vi "change_image_type.vi"(8 "error in (no error)":errorcluster, 10 "target image type":T1 items=["Grayscale (U8)", "Grayscale (I16)", "Grayscale (SGL)", "Complex (CSG)", "RGB (U32)", "HSL (U32)", "RGB (U64)", "Grayscale (U16)"], 11 "Image in":refnum<class "Image.lvclass">) -> (0 "error out":errorcluster, 3 "Image out":refnum<class "Image.lvclass">)   [LabVIEW 2010, in "Image.lvclass"]
uses:
  Image.lvclass
  storage_mode.ctl
  ErrorController/ErrorController/class_data.vi
  <vilib>/vision/NI_Vision_Development_Module.lvlib
  ErrorController/ErrorController/ErrorController.lvclass
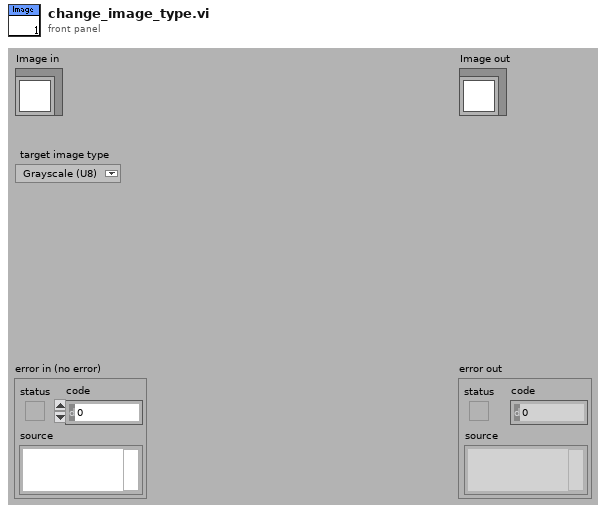
[diagram p1: front panel]
types:
  T1 = typedef "Image Type" = u32
  T2 = typedef "Image.lvclass/storage_mode.ctl" = enum16{"RAM", "disk"}
  T3 = typedef "IMAQ Image.ctl" = refnum<image>
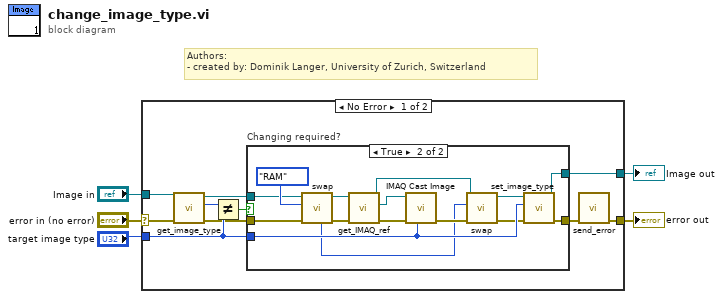
[diagram p0: block diagram]
diagram:
  # "Authors: \n- created by: Dominik Langer, University of Zurich, Switzerland"
  n1 = case shown="No Error" "error in (no error)" {
    selector: "error in (no error)" -> [w15 w34]
    tunnel: [w7 w34] -> w4
    tunnel: [w12 w33] -> w2
    tunnel: "Image in" -> [w13 w33]
    tunnel: "target image type" -> [w11 _]
    frame No Error {
      n2 = call-dynamic "get_image_type.vi"("error in (no error)"=w15, "Image.lvclass in"=w13) -> ("error out"=w10:errorcluster, "Image Type"=w14:T1, "Image.lvclass out"=w9:refnum<class "Image.lvclass">)  [unwired: 6 in, 1 out]
      n3 = Not Equal?(x=w14, y=w11) -> (x != y?=w8:bool)
      n4 = case "Changing required?" shown="True" w8 {
        tunnel: [w16 w32] -> w6
        tunnel: [w17 w29] -> w12
        tunnel: w11 -> [_ w28]
        tunnel: w10 -> [w16 w27]
        tunnel: w9 -> [w17 w24]
        frame False {
        }
        frame True {
          n5 = call-dynamic "swap.vi"("error in (no error)"=w27, "storage type target"=storage_mode."RAM", "Image in"=w24) -> ("error out"=w26:errorcluster, "Image out"=w23:refnum<class "Image.lvclass">, "previous storage mode"=w20:T2)  [unwired: 6 in]
          n6 = call-dynamic "get_IMAQ_ref.vi"("error in (no error)"=w26, "Image.lvclass in"=w23) -> ("error out"=w31:errorcluster, "Image"=w30:T3, "Image.lvclass out"=w19:refnum<class "Image.lvclass">)  [unwired: 5 in, 2 out]
          n7 = call "IMAQ Cast Image"("Image Type"=w28, "error in (no error)"=w31, "Image Src"=w30) -> ("error out"=w22:errorcluster)  [unwired: 7 in, 1 out]
          n8 = call-dynamic "swap.vi"("error in (no error)"=w22, "storage type target"=w20, "Image in"=w19) -> ("error out"=w21:errorcluster, "Image out"=w18:refnum<class "Image.lvclass">)  [unwired: 6 in, 1 out]
          n9 = call-dynamic "set_image_type.vi"("error in (no error)"=w21, "Image Type"=w28, "Image.lvclass in"=w18) -> ("error out"=w32:errorcluster, "Image.lvclass out"=w29:refnum<class "Image.lvclass">)  [unwired: 7 in]
        }
      }
      n10 = call "send_error.vi"("error in (no error)"=w6) -> ("error out"=w7:errorcluster)  [unwired: 10 in]
    }
    frame Error {
    }
  }
  "error out" <- w4
  "Image out" <- w2
